vi "convert eng. to counts.vi"(6 "Axis (1..4)":T1=1 items=["X"=1, "Y"=2, "Z"=3, "T"=4], 8 "error in (no error)":errorcluster, 9 "Position, eng units":dbl, 10 "All Positions, eng units":dbl[](array[numeric]), 11 "VXMx2 in":refnum<class "VXMx2.lvclass">) -> (0 "error out":errorcluster, 1 "Position, counts":i32, 2 "All Positions, counts":i32[](array[numeric]), 3 "VXMx2 out":refnum<class "VXMx2.lvclass">)   [LabVIEW 2018, in "VXMx2.lvclass"]
doc: "convert one position to steps.\nconvert all positions to steps."
uses:
  VXMx2.lvclass
  <instrlib>/Velmex VXM/Public/VXM Axis.ctl
  VXMx2.lvclass/VXMx2.ctl
  <instrlib>/Velmex VXM/Velmex VXM.lvlib
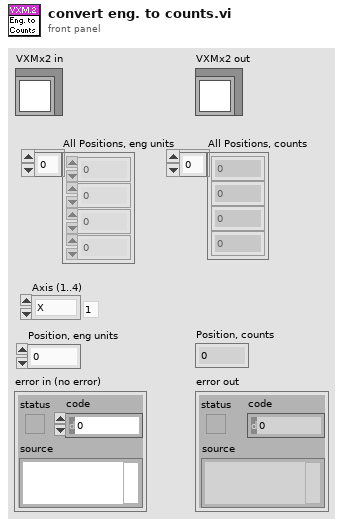
[diagram p1: front panel]
types:
  T1 = typedef "Velmex VXM.lvlib/VXM Axis.ctl" = u16
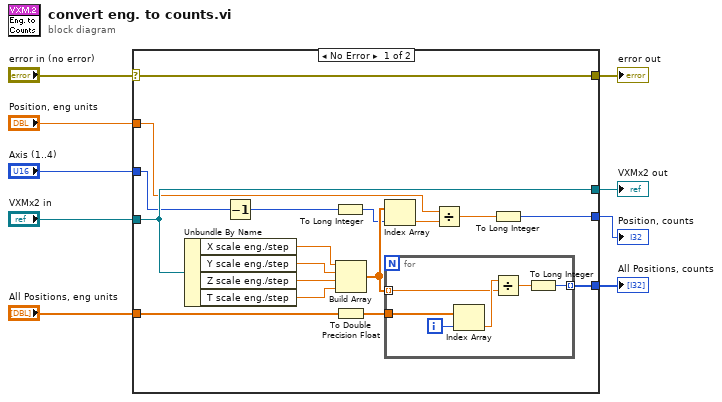
[diagram p0: block diagram]
diagram:
  n1 = case shown="No Error" "error in (no error)" {
    selector: "error in (no error)" -> [w26 w34]
    tunnel: [w26 w34] -> w8
    tunnel: [w25 w33] -> w6
    tunnel: "VXMx2 in" -> [w25 w33]
    tunnel: "All Positions, eng units" -> [w20 _]
    tunnel: [w18 _] -> w4
    tunnel: "Axis (1..4)" -> [w16 _]
    tunnel: "Position, eng units" -> [w11 _]
    tunnel: [w10 _] -> w1
    frame No Error {
      n2 = Unbundle By Name(w25) -> ("X scale eng./step"=w24:dbl, "Y scale eng./step"=w23:dbl, "Z scale eng./step"=w22:dbl, "T scale eng./step"=w21:dbl)
      n3 = Decrement(x=w16) -> (x-1=w15:T1)
      n4 = To Long Integer(number=w15) -> (32bit integer=w14:i32)
      n5 = Build Array(w24, w23, w22, w21) -> (w17:dbl[])
      n6 = To Double Precision Float(number=w20) -> (double precision float=w19:dbl[])
      n7 = Index Array(array=w17, index=w14) -> (element=w13:dbl)
      n8 = for {
        tunnel: w17 -> [w28] mode=indexing
        tunnel: w19 -> [w31]
        tunnel: [w27] -> w18 mode=indexing
        i -> [w32]
        n9 = Index Array(array=w31, index=w32) -> (element=w29:dbl)
        n10 = Divide(x=w29, y=w28) -> (x/y=w30:dbl)
        n11 = To Long Integer(number=w30) -> (32bit integer=w27:i32)
      }
      n12 = Divide(x=w11, y=w13) -> (x/y=w12:dbl)
      n13 = To Long Integer(number=w12) -> (32bit integer=w10:i32)
    }
    frame Error {
    }
  }
  "error out" <- w8
  "VXMx2 out" <- w6
  "All Positions, counts" <- w4
  "Position, counts" <- w1
